vi "FTW-Ether-Tag-Construct.vi"(5 "FTW Ether Configuration":string="{\n  \"ApplicationName\": \"Featherweight Application\",\n  \"ApplicationVersion\": \"0.1.0-1\",\n  \"LoggerAddress\": \"inproc://*\",\n  \"LoggerName\": \"Log\",\n  \"LoggerDirectory\": \"[UserAppData]\\\\Featherweight\\\\Logs\",\n  \"LoggerDiskThrashDelay\": 200\n}", 11 "error in":errorcluster) -> (15 "error out":errorcluster)   [LabVIEW 2015, in "FTW-Ether.lvclass"]
uses:
  FTW-Ether.lvclass
  JSON/FTW-JSON-JoinMode.ctl
  FTW-Ether-Instance.vi
  container/FTW-Container.lvclass
panel:
  # "Inputs"
  # "Outputs"
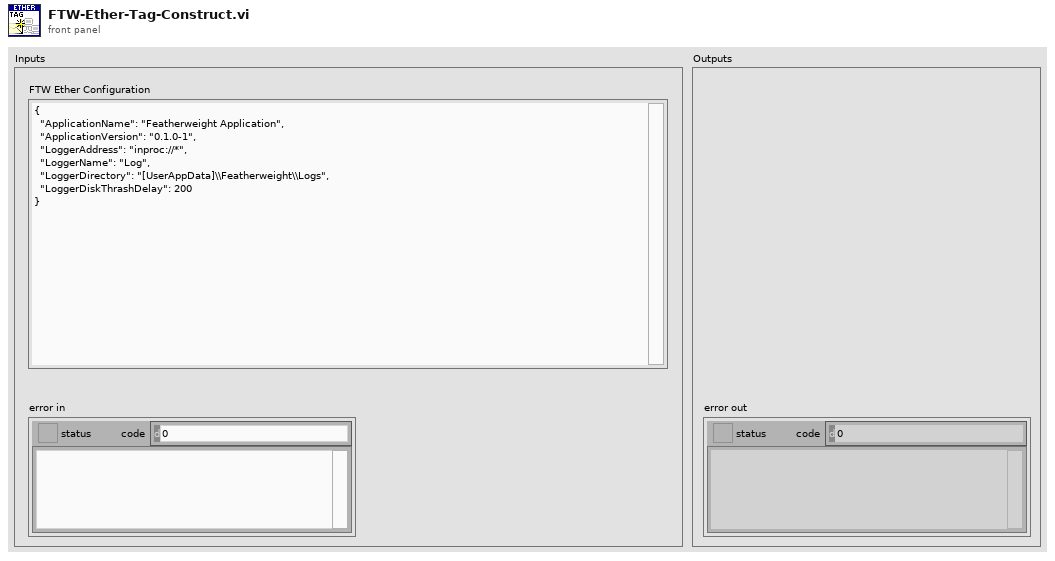
[diagram p1: front panel]
types:
  T1 = typedef "FTW-JSON-JoinMode.ctl" = enum32{"Upsert", "Update Only", "Insert Only"}
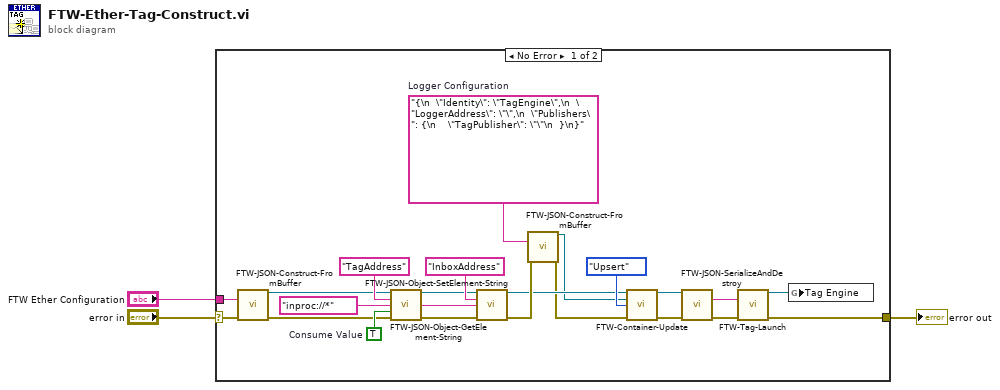
[diagram p0: block diagram]
diagram:
  n1 = case shown="No Error" "error in" {
    selector: "error in" -> [w26 w27]
    tunnel: [w25 w27] -> w1
    tunnel: "FTW Ether Configuration" -> [w13 _]
    frame No Error {
      w7 = "{\n  \"Identity\": \"TagEngine\",\n  \"LoggerAddress\": \"\",\n  \"Publishers\": {\n    \"TagPublisher\": \"\"\n  }\n}"  # Logger Configuration
      w18 = TRUE  # Consume Value
      n2 = call "FTW-JSON-Construct-FromBuffer.vi"("JSON String (UTF-8)"=w13, "error in"=w26) -> ("JSON"=w12:refnum<class "FTW-Container.lvclass">, "error out"=w14:errorcluster)  [unwired: 12 in]
      n3 = call "FTW-JSON-Object-GetElement-String.vi"("JSON"=w12, "Key"="TagAddress", "Default Value"="inproc://*", "Consume Value"=w18, "error in"=w14) -> ("JSON out"=w11:refnum<class "FTW-Container.lvclass">, "Value"=w16:string, "error out"=w21:errorcluster)  [unwired: 6 in, 2 out]
      n4 = call "FTW-JSON-Object-SetElement-String.vi"("JSON"=w11, "Key"="InboxAddress", "Value"=w16, "error in"=w21) -> ("JSON out"=w10:refnum<class "FTW-Container.lvclass">, "error out"=w17:errorcluster)  [unwired: 10 in]
      n5 = call "FTW-JSON-Construct-FromBuffer.vi"("JSON String (UTF-8)"=w7, "error in"=w17) -> ("JSON"=w8:refnum<class "FTW-Container.lvclass">, "error out"=w9:errorcluster)  [unwired: 12 in]
      n6 = call "FTW-Container-Update.vi"("FTW-Container In"=w10, "Other Container"=w8, "Join Mode"=FTW-JSON-JoinMode."Upsert" ("Update Mode (0: Upsert)"), "error in"=w9) -> ("Updated Container"=w5:refnum<class "FTW-Container.lvclass">, "error out"=w23:errorcluster)  [unwired: 10 in]
      n7 = call "FTW-JSON-SerializeAndDestroy.vi"("JSON"=w5, "error in"=w23) -> ("JSON String (UTF-8)"=w4:string, "error out"=w6:errorcluster)  [unwired: 12 in]
      n8 = call "FTW-Tag-Launch.vi"("FTW Tag Configuration"=w4, "error in"=w6) -> ("FTW Tag Connector"=w24:refnum<class "FTW-ActorConnector.lvclass">, "error out"=w25:errorcluster)  [unwired: 10 in, 2 out]
      n9 = global write "FTW-Ether-Instance.vi" "Tag Engine"(w24) -> ()
    }
    frame Error {
    }
  }
  "error out" <- w1
